vi "M_TestPath.vi"() -> ()   [LabVIEW 2016]
panel:
  out "VI路径":path
  in  "布尔":bool
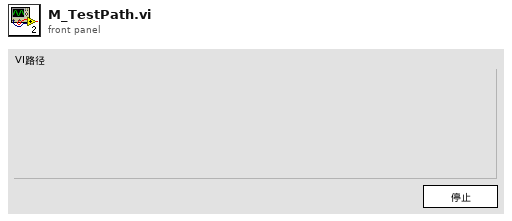
[diagram p1: front panel]
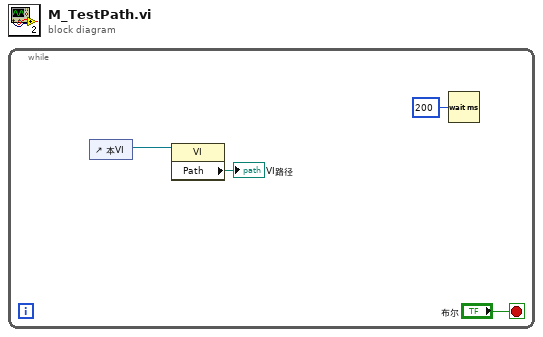
[diagram p0: block diagram]
diagram:
  n1 = while {
    stop <- "布尔" stop-if-true
    n2 = control-ref of="本VI"() -> (w4:refnum<vi>)
    n3 = property class="VI"(reference=w4) -> ("Path"=→"VI路径":path)  [unwired: 1 in, 2 out]
    n4 = Wait (ms)(milliseconds to wait=u32 200 ("等待时间（毫秒）")) -> ()  [unwired: 1 out]
  }
